vi "mod_check.vi"(5 "connection reference":T3) -> ()   [LabVIEW 2018]
uses:
  <vilib>/addons/database/Connection.llb/Conn ObjectReference.ctl
  <vilib>/addons/database/Connection.llb/Conn Execute.vi
  <vilib>/addons/database/Recordset.llb/Rec Fetch Recordset Data (R).vi
  <vilib>/addons/database/_DB Variant To Data/Database Variant To Data.xnode
  <vilib>/addons/database/NI_Database_API.lvlib
panel:
  out "字符串":string
  in  "日期格式化显示":string="%Y-%m-%d"
  in  "表名":string="room_check"
  in  "表字段类型簇":T1
  out "数组":string[](array[string])
  in  "字段名数组":string[](array[string])=["apartmentNamegyc", "roomIDgyc", "timegyc", "situationgyc", ""]
  out "error out":errorcluster
  in  "修改按钮":bool
  in  "清除指示灯":bool
  in  "添加按钮":bool
  in  "删除按钮":bool
  in  "查询按钮":bool
  in  "信息输入框":T2
  in  "刷新按钮":bool
  in  "信息框":i32(listbox)
  in  "已编辑行数组":u32[](array[numeric])
  in  "信息框缓冲备份":string[][](array[string])
  in  "error in (no error)":errorcluster
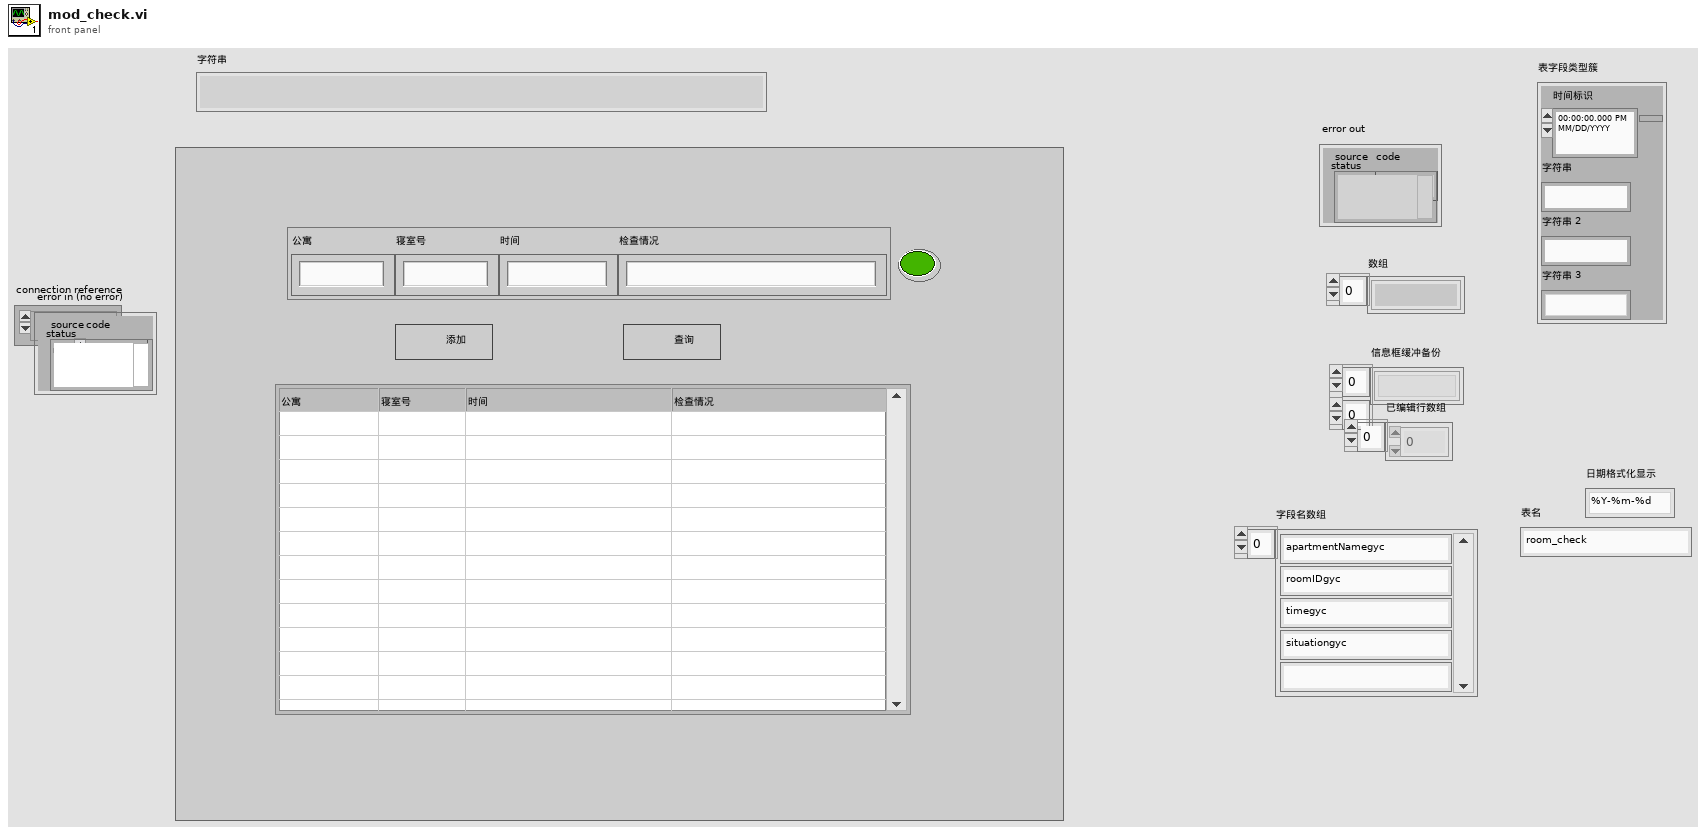
[diagram p1: front panel]
types:
  T1 = cluster{"时间标识":timestamp, "字符串":string, "字符串 2":string, "字符串 3":string}
  T2 = cluster{"公寓":string, "寝室号":string, "时间":string, "检查情况":string}
  T3 = typedef "NI_Database_API.lvlib/Conn ObjectReference.ctl" = refnum<k1>
  T4 = typedef "LVPoint32TypeDef.ctl" = cluster{"Horizontal":i32, "Vertical":i32}
  T5 = typedef "LVRowAndColumnTypeDef.ctl" = cluster{"Row":i32, "Column":i32}
  T6 = typedef "NI_Database_API.lvlib/Rec ObjectReference.ctl" = refnum<k1>
  T7 = cluster{"[0]":string, "[1]":string, "[2]":string, "[3]":string}
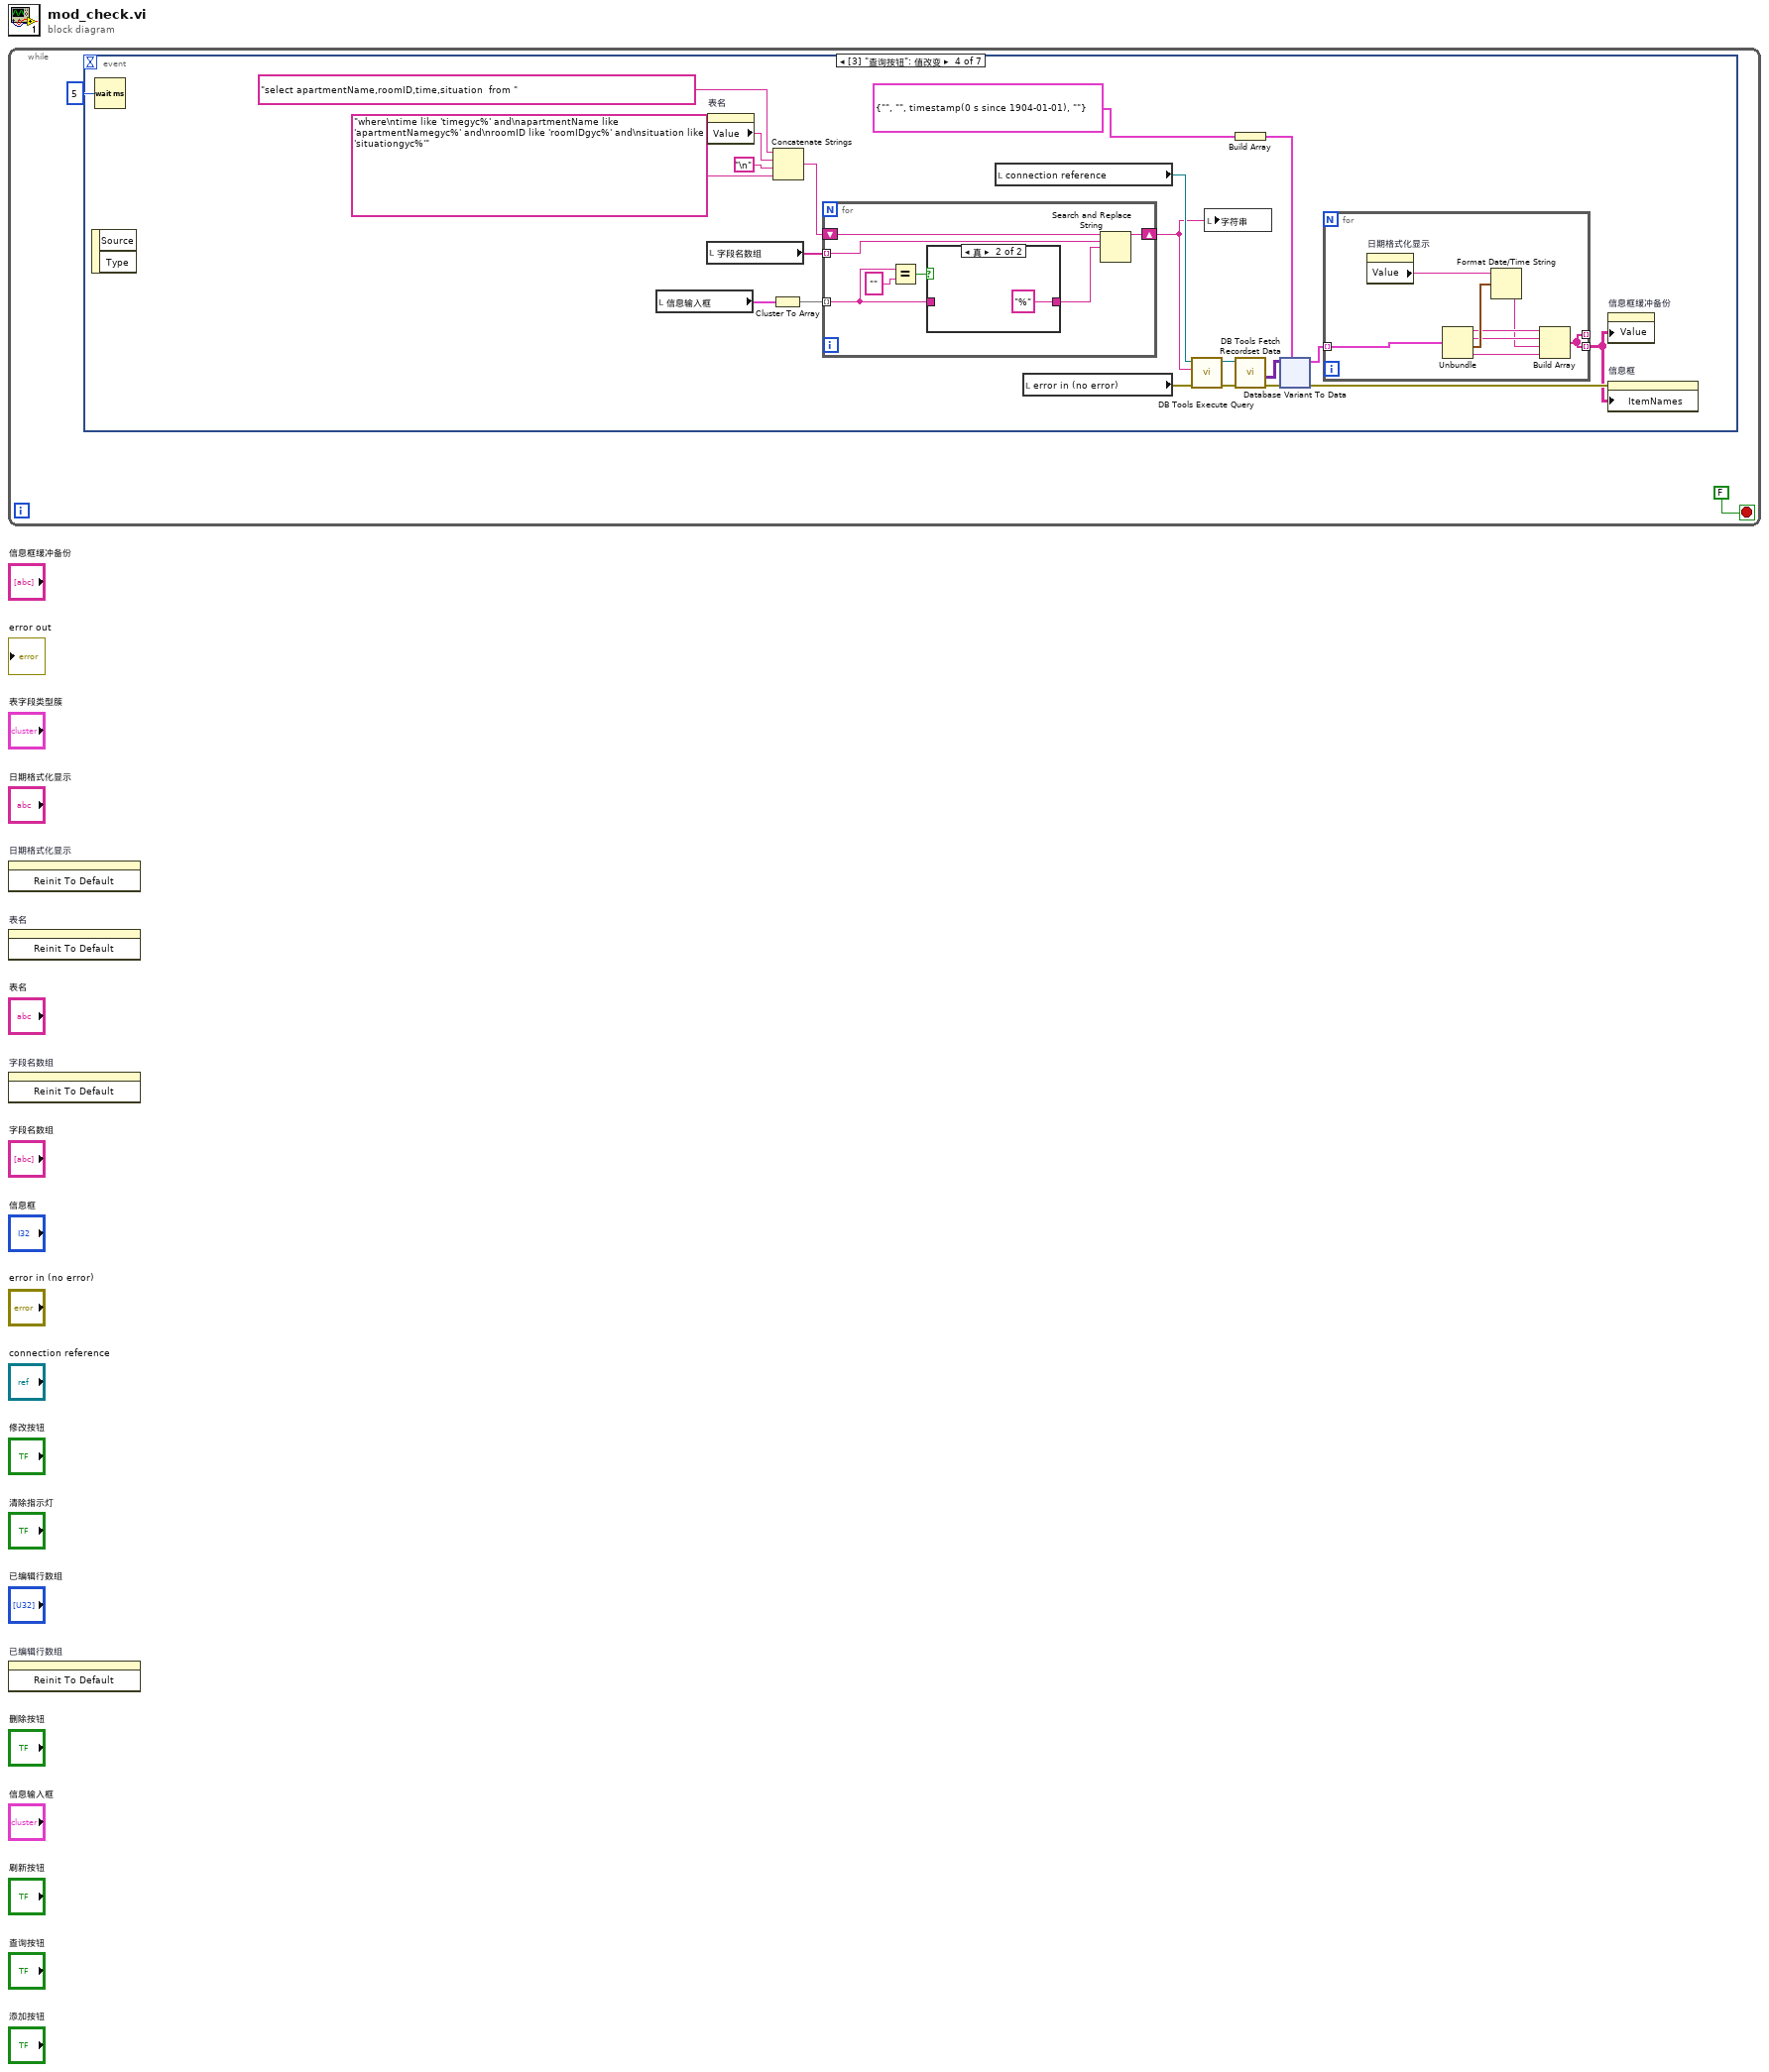
[diagram p0: block diagram]
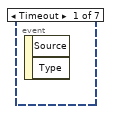
[diagram p2: hidden frame]
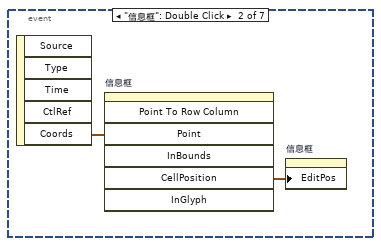
[diagram p3: hidden frame]
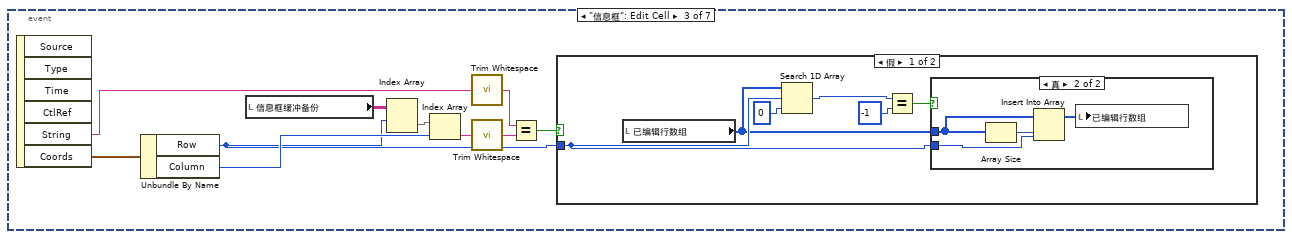
[diagram p4: hidden frame]
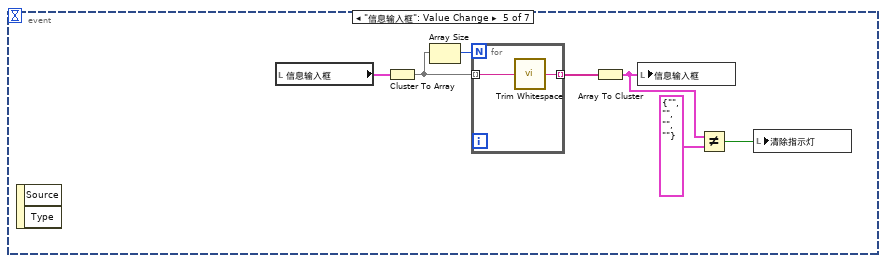
[diagram p8: hidden frame]
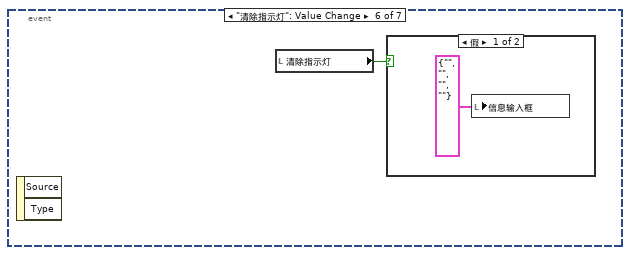
[diagram p9: hidden frame]
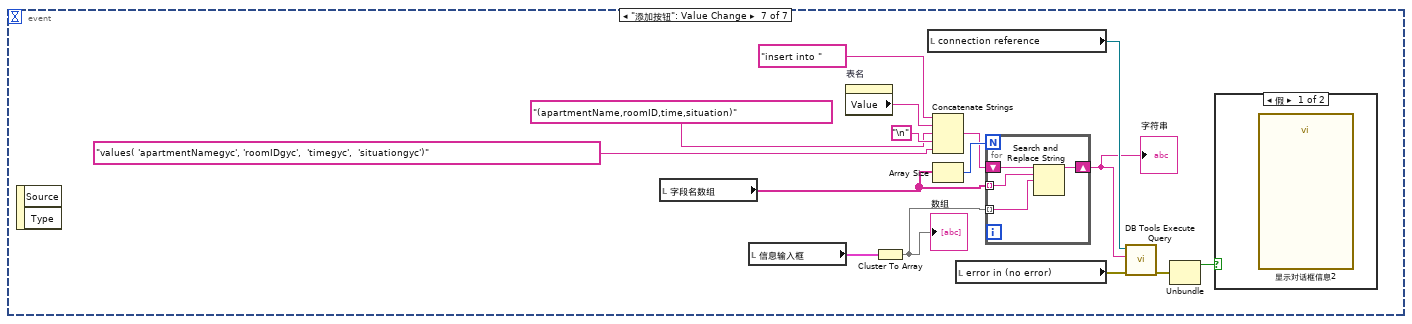
[diagram p11: hidden frame]
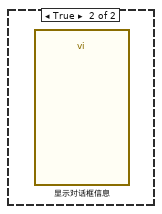
[diagram p12: hidden frame]
diagram:
  n1 = while {
    stop <- FALSE stop-if-true
    n2 = event shown="[3] \"查询按钮\": 值改变" {
      selector: _ -> [_ _ _ _ _ _ _]
      dyn-events: _ -> [_ _ _ _ _ _ _]
      timeout: _ -> [_ _ _ _ _ _ _]
      event Timeout {
        n3 = event-data() -> ()  [unwired: 1 in, 2 out]
      }
      event "信息框": Double Click {
        n4 = event-data() -> ("Coords"=w4:T4)  [unwired: 1 in, 4 out]
        n5 = invoke on="信息框" class="MCListbox (严格)" method="Point To Row Column"("Point"=w4) -> ("CellPosition"=w3:T5)  [unwired: 6 in, 6 out]
        n6 = property on="信息框" class="MCListbox (严格)"("EditPos"=w3) -> ()  [unwired: 2 in, 2 out]
      }
      event "信息框": Edit Cell {
        n7 = event-data() -> ("String"=w9:string, "Coords"=w10:T5)  [unwired: 1 in, 4 out]
        n8 = Unbundle By Name(w10) -> ("Row"=w12:i32, "Column"=w14:i32)
        n9 = local read "信息框缓冲备份"() -> (w11:string[][])
        n10 = Index Array(array=w11, index (row)=w12) -> (element=w13:string[])  [unwired: 1 in]
        n11 = Index Array(array=w13, index=w14) -> (element=w7:string)
        n12 = call <vilib>:"Trim Whitespace.vi"("string"=w9) -> ("trimmed string"=w8:string)  [unwired: 1 in]
        n13 = call <vilib>:"Trim Whitespace.vi"("string"=w7) -> ("trimmed string"=w6:string)  [unwired: 1 in]
        n14 = Equal?(x=w8, y=w6) -> (x = y?=w5:bool)
        n15 = case shown="假" w5 {
          tunnel: w12 -> [w20 _]
          frame False {
            n16 = local read "已编辑行数组"() -> (w18:u32[])
            n17 = Search 1D Array(1D array=w18, element=w20, start index (0)=0 ("开始索引(0)")) -> (index of element=w19:i32)
            n18 = Equal?(x=w19, y=-1) -> (x = y?=w17:bool)
            n19 = case shown="真" w17 {
              tunnel: w18 -> [_ w22]
              tunnel: w20 -> [_ w24]
              frame False {
              }
              frame True {
                n20 = Array Size(array=w22) -> (size(s)=w21:i32)
                n21 = Insert Into Array(array=w22, index=w21, new element=w24) -> (w23:u32[])
                n22 = local write "已编辑行数组"(w23) -> ()
              }
            }
          }
          frame True {
          }
        }
      }
      event "查询按钮": Value Change {
        n23 = event-data() -> ()  [unwired: 1 in, 2 out]
        n24 = local read "信息输入框"() -> (w35:T2)
        n25 = local read "字段名数组"() -> (w33:string[])
        n26 = property on="表名" class="Str"() -> ("Value"=w31:string)  [unwired: 2 in, 2 out]
        n27 = Cluster To Array(cluster=w35) -> (array=w34:string[])
        n28 = Concatenate Strings("select apartmentName,roomID,time,situation  from ", w31, "\n", "where\ntime like 'timegyc%' and\napartmentName like 'apartmentNamegyc%' and\nroomID like 'roomIDgyc%' and\nsituation like 'situationgyc%'") -> (w32:string)
        n29 = for {
          shift-right: [w50] -> w25
          shift-left: w32 -> [w51]
          tunnel: w33 -> [w47] mode=indexing
          tunnel: w34 -> [w46] mode=indexing
          n30 = Equal?(x=w46, y="") -> (x = y?=w49:bool)
          n31 = case shown="真" w49 {
            tunnel: [w52 "%"] -> w45
            tunnel: w46 -> [w52 _]
            frame False {
            }
            frame True {
            }
          }
          n32 = Search and Replace String(input string=w51, search string=w47, replace string=w45) -> (result string=w50:string)  [unwired: 5 in, 3 out]
        }
        n33 = local read "connection reference"() -> (w44:T3)
        n34 = local read "error in (no error)"() -> (w43:errorcluster)
        n35 = call-poly <vilib>:"DB Tools Execute Query.vi"("error in (no error)"=w43, "SQL query"=w25, "connection reference"=w44) -> ("error out"=w36:errorcluster, "recordset reference"=w37:T6)  [unwired: 5 in]
        n36 = local write "字符串"(w25) -> ()
        n37 = Build Array(cluster{string, string, timestamp, string} {"", "", timestamp(0 s since 1904-01-01), ""}) -> (w40:cluster{string, string, timestamp, string}[])
        n38 = call-poly <vilib>:"DB Tools Fetch Recordset Data.vi"("error in (no error)"=w36, "recordset reference"=w37) -> ("error out"=w38:errorcluster, "recordset data"=w39:variant[][])  [unwired: 3 in, 1 out]
        n39 = xnode "Database Variant To Data"("database variant"=w39, "error in (no error)"=w38, "type"=w40) -> ("data"=w41:cluster{string, string, timestamp, string}[], "error out"=w42:errorcluster)
        n40 = for {
          tunnel: w41 -> [w61] mode=indexing
          tunnel: [w59] -> _ mode=indexing
          tunnel: [w59] -> w27 mode=indexing
          n41 = property on="日期格式化显示" class="Str"() -> ("Value"=w60:string)  [unwired: 2 in, 2 out]
          n42 = Unbundle(w61) -> (w56:string, w55:string, w57:timestamp, w58:string)
          n43 = Format Date/Time String(time format string (%c)=w60, seconds (now)=w57) -> (date/time string=w54:string)  [unwired: 1 in]
          n44 = Build Array(w56, w55, w54, w58) -> (w59:string[])
        }
        n45 = property on="信息框缓冲备份" class="Arr (严格)"("Value"=w27) -> ()  [unwired: 2 in, 2 out]
        n46 = property on="信息框" class="MCListbox (严格)"(error in=w42, "ItemNames"=w27) -> ()  [unwired: 1 in, 2 out]
      }
      event "信息输入框": Value Change {
        n47 = event-data() -> ()  [unwired: 1 in, 2 out]
        n48 = local read "信息输入框"() -> (w212:T2)
        n49 = Cluster To Array(cluster=w212) -> (array=w211:string[])
        n50 = Array Size(array=w211) -> (size(s)=w213:i32)
        n51 = for {
          N: w213 -> [_]
          tunnel: w211 -> [w217] mode=indexing
          tunnel: [w216] -> w210 mode=indexing
          n52 = call <vilib>:"Trim Whitespace.vi"("string"=w217) -> ("trimmed string"=w216:string)  [unwired: 1 in]
        }
        n53 = Array To Cluster(array=w210) -> (cluster=w209:T7)
        n54 = local write "信息输入框"(w209) -> ()
        n55 = Not Equal?(x=w209, y=cluster{string, string, string, string} {"", "", "", ""}) -> (x != y?=w214:bool)
        n56 = local write "清除指示灯"(w214) -> ()
      }
      event "清除指示灯": Value Change {
        n57 = event-data() -> ()  [unwired: 1 in, 2 out]
        n58 = local read "清除指示灯"() -> (w218:bool)
        n59 = case shown="假" w218 {
          frame False {
            n60 = local write "信息输入框"(cluster{string, string, string, string} {"", "", "", ""}) -> ()
          }
          frame True {
          }
        }
      }
      event "添加按钮": Value Change {
        n61 = event-data() -> ()  [unwired: 1 in, 2 out]
        n62 = local read "字段名数组"() -> (w227:string[])
        n63 = local read "信息输入框"() -> (w229:T2)
        n64 = property on="表名" class="Str"() -> ("Value"=w224:string)  [unwired: 2 in, 2 out]
        n65 = Cluster To Array(cluster=w229) -> (array=w228:string[])
        "数组" <- w228
        n66 = local read "connection reference"() -> (w233:T3)
        n67 = Concatenate Strings("insert into " ("SQL query"), w224, "(apartmentName,roomID,time,situation)", "\n", "values( 'apartmentNamegyc', 'roomIDgyc',  'timegyc',  'situationgyc')") -> (w226:string)
        n68 = Array Size(array=w227) -> (size(s)=w230:i32)
        n69 = local read "error in (no error)"() -> (w234:errorcluster)
        n70 = for {
          N: w230 -> [_]
          shift-right: [w238] -> w220
          shift-left: w226 -> [w237]
          tunnel: w228 -> [w236] mode=indexing
          tunnel: w227 -> [w235] mode=indexing
          n71 = Search and Replace String(input string=w237, search string=w235, replace string=w236) -> (result string=w238:string)  [unwired: 5 in, 3 out]
        }
        "字符串" <- w220
        n72 = call-poly <vilib>:"DB Tools Execute Query.vi"("error in (no error)"=w234, "SQL query"=w220, "connection reference"=w233) -> ("error out"=w232:errorcluster)  [unwired: 5 in, 1 out]
        n73 = Unbundle(w232) -> ("status"=w231:bool)  [unwired: 2 out]
        n74 = case shown="假" w231 {
          frame False {
            n75 = call "显示对话框信息2"() -> ()  [unwired: 10 in, 2 out]
          }
          frame True {
            n76 = call "显示对话框信息"() -> ()  [unwired: 10 in, 2 out]
          }
        }
      }
    }
    n77 = Wait (ms)(milliseconds to wait=u32 5 ("等待时间（毫秒）")) -> ()  [unwired: 1 out]
  }
  n78 = invoke on="日期格式化显示" class="Str" method="Reinit To Default"() -> ()  [unwired: 3 in, 3 out]
  n79 = invoke on="表名" class="Str" method="Reinit To Default"() -> ()  [unwired: 3 in, 3 out]
  n80 = invoke on="字段名数组" class="Arr (严格)" method="Reinit To Default"() -> ()  [unwired: 3 in, 3 out]
  n81 = invoke on="已编辑行数组" class="Arr (严格)" method="Reinit To Default"() -> ()  [unwired: 3 in, 3 out]
